vi "hse-application_DetermineAppBasePath.vi"(8 "error in (no error)":errorcluster, 10 "Application Directory":path) -> (0 "error out":errorcluster, 2 "Application Directory DUP":path, 3 "App Base Path":path)   [LabVIEW 2014, in "hse-application.lvclass"]
doc: "Determines the \"Root\" path of the application: \n- When running from the development environment, this is identical to the application directory. \n- When running from the run-time environment, this includes the name of the .exe"
uses:
  hse-application.lvclass
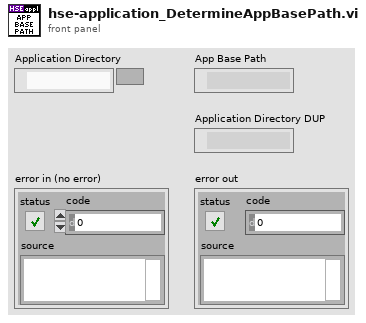
[diagram p1: front panel]
types:
  T1 = enum32{"invalid app kind", "Development System", "Run Time System", "Student Edition", "Embedded LabVIEW", "Evaluation", "Custom"}
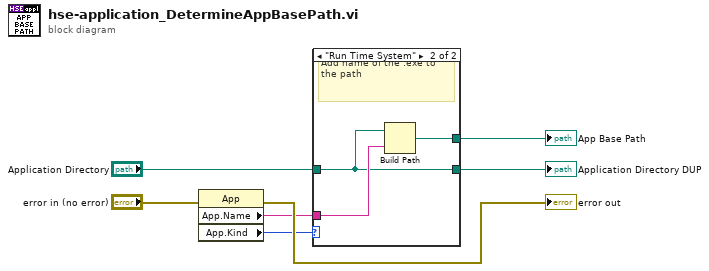
[diagram p0: block diagram]
diagram:
  n1 = property class="App"(error in="error in (no error)") -> (error out=→"error out":errorcluster, "App.Name"=w2:string, "App.Kind"=w5:T1)  [unwired: 1 in, 1 out]
  n2 = case shown="\"Run Time System\"" w5 {
    tunnel: "Application Directory" -> [w8 w9]
    tunnel: [w8 w11] -> w4
    tunnel: w2 -> [_ w10]
    tunnel: [w8 w9] -> w1
    frame Default {
      # "Base path = Application Directory"
    }
    frame "Run Time System" {
      # "Add name of the .exe to the path"
      n3 = Build Path(base path=w9, name or relative path=w10) -> (appended path=w11:path)
    }
  }
  "App Base Path" <- w4
  "Application Directory DUP" <- w1
